vi "Git-Extract Page Numbers from Header Link.vi"(11 "Link":string) -> (2 "Pages":string, 3 "Current Page":string)   [LabVIEW 2020]
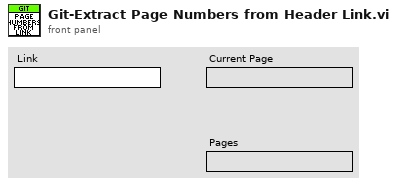
[diagram p1: front panel]
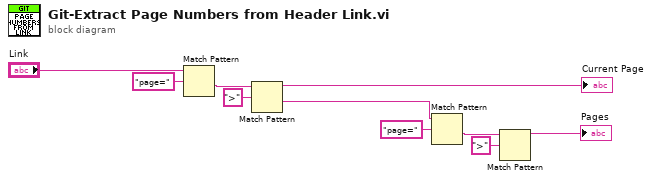
[diagram p0: block diagram]
diagram:
  n1 = Match Pattern(string="Link", regular expression="page=") -> (after substring=w4:string)  [unwired: 1 in, 3 out]
  n2 = Match Pattern(string=w4, regular expression=">") -> (before substring=→"Current Page":string, after substring=w9:string)  [unwired: 1 in, 2 out]
  n3 = Match Pattern(string=w9, regular expression="page=") -> (after substring=w6:string)  [unwired: 1 in, 3 out]
  n4 = Match Pattern(string=w6, regular expression=">") -> (before substring=→"Pages":string)  [unwired: 1 in, 3 out]
